vi "Format XY Plot.vi"(4 "Active Y Scale (Left or Right)":u32[](array[numeric]), 6 "Line Styles":u8[](array[numeric]), 8 "Plot Interpolation":u8=2, 9 "Colors Array":u32[](array[colorbox])=[16711680, 13434624, 65382, 26111, 13435135], 10 "Plot Names":string[](array[string]), 11 "XY Graph Reference":refnum<vi>) -> ()   [LabVIEW 2010]
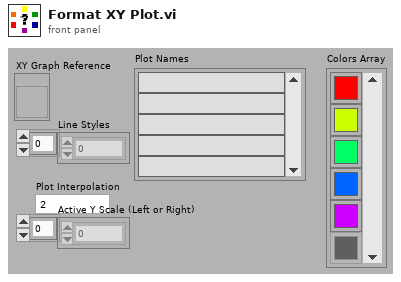
[diagram p1: front panel]
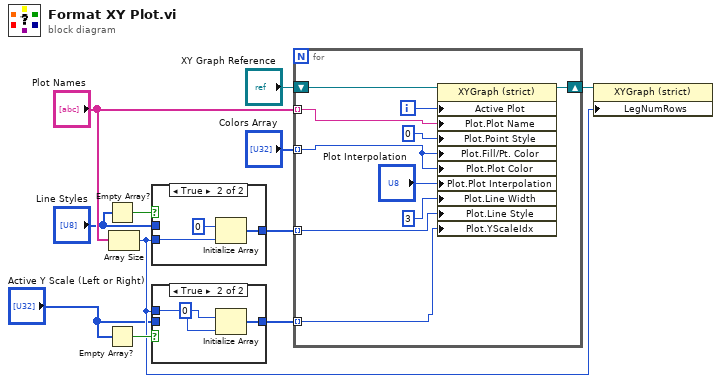
[diagram p0: block diagram]
diagram:
  n1 = Empty Array?(array="Line Styles") -> (empty?=w7:bool)
  n2 = Empty Array?(array="Active Y Scale (Left or Right)") -> (empty?=w4:bool)
  n3 = Array Size(array="Plot Names") -> (size(s)=w3:i32)
  n4 = case shown="True" w7 {
    tunnel: "Line Styles" -> [w12 _]
    tunnel: [w12 w13] -> w5
    tunnel: w3 -> [_ w15]
    frame False {
    }
    frame True {
      n5 = Initialize Array(u8 0 ("Plot.Line Style"), w15) -> (w13:u8[])
    }
  }
  n6 = case shown="True" w4 {
    tunnel: "Active Y Scale (Left or Right)" -> [w16 _]
    tunnel: [w16 w18] -> w1
    tunnel: w3 -> [_ w19]
    frame False {
    }
    frame True {
      n7 = Initialize Array(u32 0 ("Plot.Y Scale Index"), w19) -> (w18:u32[])
    }
  }
  n8 = for {
    shift-right: [w28] -> w10
    shift-left: "XY Graph Reference" -> [w29]
    tunnel: "Plot Names" -> [w26] mode=indexing
    tunnel: "Colors Array" -> [w24] mode=indexing
    tunnel: w5 -> [w21] mode=indexing
    tunnel: w1 -> [w20] mode=indexing
    i -> [w27]
    n9 = property on="Property Node" class="XYGraph (strict)"(reference=w29, "Active Plot"=w27, "Plot.Plot Name"=w26, "Plot.Point Style"=u8 0, "Plot.Fill/Pt. Color"=w24, "Plot.Plot Color"=w24, "Plot.Plot Interpolation"="Plot Interpolation", "Plot.Line Width"=u8 3, "Plot.Line Style"=w21, "Plot.YScaleIdx"=w20) -> (reference out=w28:refnum<vi>)  [unwired: 1 in, 1 out]
  }
  n10 = property on="Property Node" class="XYGraph (strict)"(reference=w10, "LegNumRows"=w3) -> ()  [unwired: 1 in, 2 out]
